vi "res_calc.vi"() -> ()   [LabVIEW 2020]
panel:
  out "Array 2":dbl[](array[numeric])
  out "Array":dbl[](array[numeric])
  out "second subarray":dbl[](array[numeric])
  out "first subarray":dbl[](array[numeric])
  in  "Res":dbl[](array[numeric])
  in  "Input V":dbl
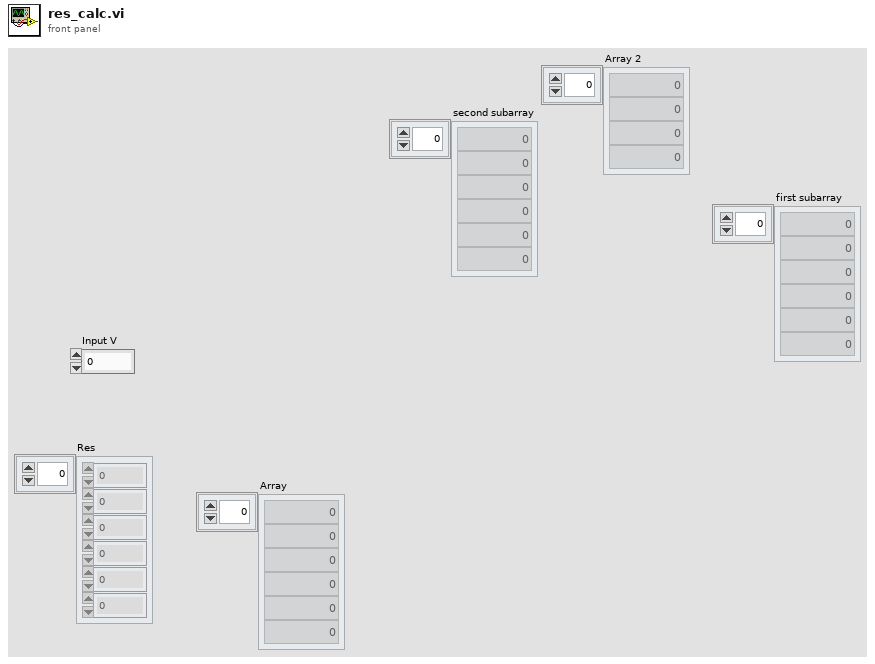
[diagram p1: front panel]
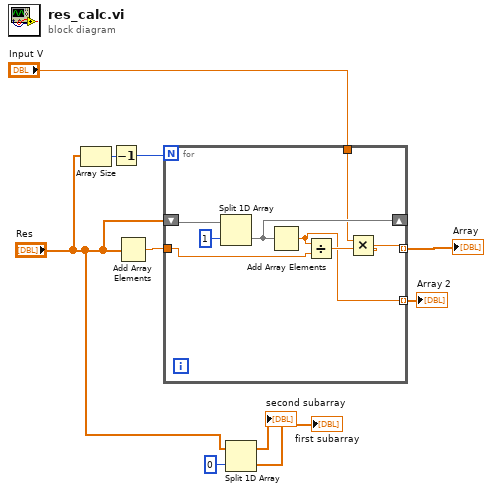
[diagram p0: block diagram]
diagram:
  n1 = Array Size(array="Res") -> (size(s)=w3:i32)
  n2 = Decrement(x=w3) -> (x-1=w1:i32)
  n3 = Add Array Elements(numeric array="Res") -> (sum=w10:dbl)
  n4 = for {
    N: w1 -> [_]
    tunnel: w10 -> [w17]
    tunnel: [w13] -> w5 mode=indexing
    shift-right: [w16] -> _
    shift-left: "Res" -> [w18]
    tunnel: "Input V" -> [w14]
    tunnel: [w12] -> w2 mode=indexing
    n5 = Split 1D Array(array=w18, index=1) -> (second subarray=w16:dbl[])  [unwired: 1 out]
    n6 = Add Array Elements(numeric array=w16) -> (sum=w12:dbl)
    n7 = Divide(x=w12, y=w17) -> (x/y=w15:dbl)
    n8 = Multiply(x=w14, y=w15) -> (x*y=w13:dbl)
  }
  "Array" <- w5
  "Array 2" <- w2
  n9 = Split 1D Array(array="Res", index=0) -> (first subarray=→"first subarray":dbl[], second subarray=→"second subarray":dbl[])
